vi "CS Active.vi"(7 "SPI Peripheral in":refnum<class "SPI Peripheral.lvclass">, 8 "error in (no error)":errorcluster, 10 "CS Active":bool, 11 "Session In":refnum<class "Session.lvclass">) -> (0 "error out":errorcluster, 3 "Session Out":refnum<class "Session.lvclass">)   [LabVIEW 2020, in "CTI.lvlib" / "SPI Peripheral.lvclass"]
uses:
  SPI Peripheral.lvclass
  Session/Session.lvclass
  SPI Peripheral.lvclass/SPI Peripheral.ctl
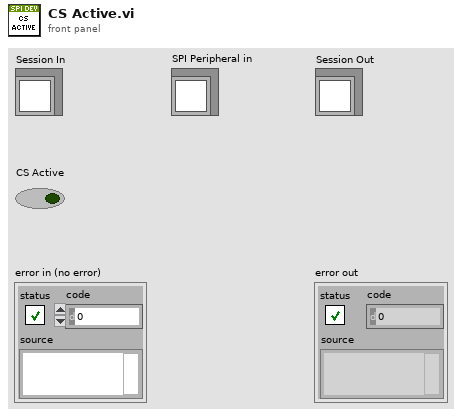
[diagram p1: front panel]
types:
  T1 = typedef "CTI.lvlib/GPIO Number.ctl" = i8
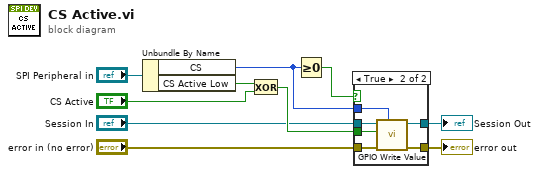
[diagram p0: block diagram]
diagram:
  n1 = Unbundle By Name("SPI Peripheral in") -> ("CS"=w9:T1, "CS Active Low"=w7:bool)
  n2 = Exclusive Or(1:"CS Active", 2:w7) -> (0:w5:bool)
  n3 = Greater Or Equal To 0?(x=w9) -> (x >= 0?=w10:bool)
  n4 = case shown="True" w10 {
    tunnel: [w11 w18] -> w2
    tunnel: [w12 w17] -> w3
    tunnel: w9 -> [_ w16]
    tunnel: w5 -> [_ w15]
    tunnel: "Session In" -> [w12 w14]
    tunnel: "error in (no error)" -> [w11 w13]
    frame False {
    }
    frame True {
      n5 = call "GPIO Write Value.vi"("GPIO #"=w16, "error in (no error)"=w13, "Value"=w15, "Session in"=w14) -> ("error out"=w18:errorcluster, "Session out"=w17:refnum<class "Session.lvclass">)  [unwired: 6 in]
    }
  }
  "error out" <- w2
  "Session Out" <- w3
